vi "sub_UDP_Transmit.vi"(7 "UDP Config":T1, 8 "error in":errorcluster, 10 "Packets":string[](array[string]), 11 "UDP Network Connection in":refnum<k16>) -> (0 "error out":errorcluster, 3 "UDP Network Connection out":refnum<k16>)   [LabVIEW 2012]
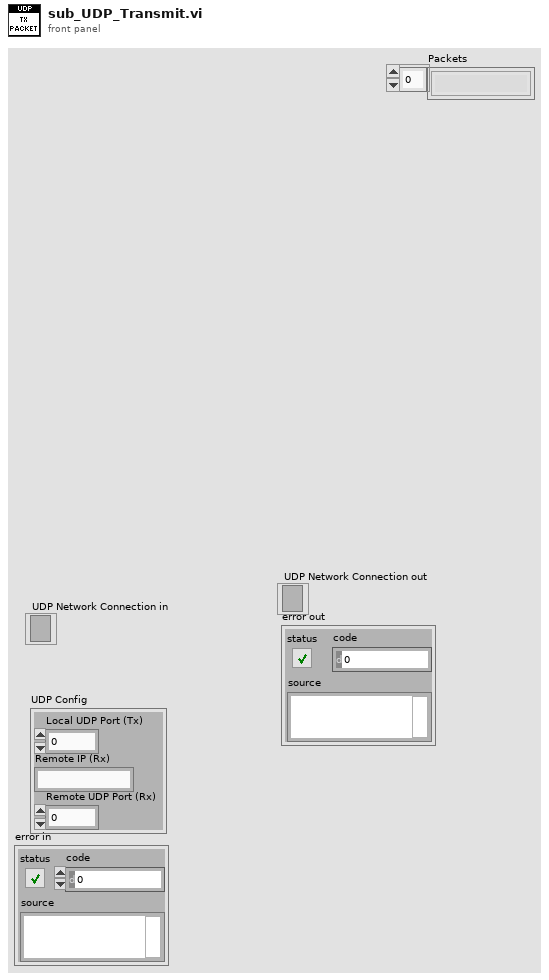
[diagram p1: front panel]
types:
  T1 = cluster{"Local UDP Port (Tx)":i16, "Remote IP (Rx)":string, "Remote UDP Port (Rx)":i16}
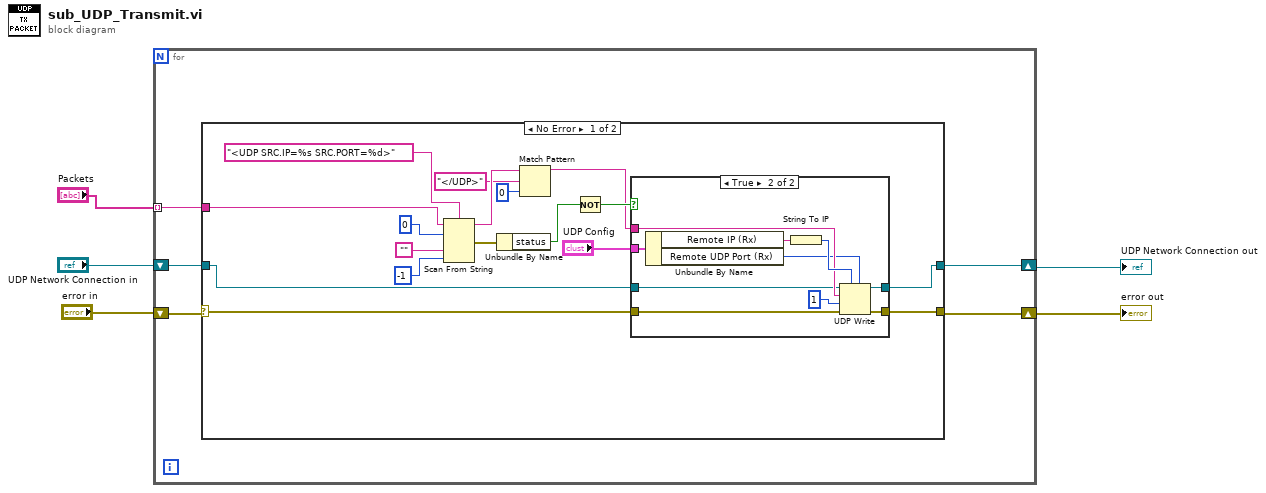
[diagram p0: block diagram]
diagram:
  n1 = for {
    shift-right: [w9] -> w4
    shift-left: "error in" -> [w7]
    shift-right: [w10] -> w5
    shift-left: "UDP Network Connection in" -> [w8]
    tunnel: "Packets" -> [w6] mode=indexing
    n2 = case shown="No Error" w7 {
      selector: w7 -> [w17 w41]
      tunnel: [w19 w40] -> w10
      tunnel: [w18 w41] -> w9
      tunnel: w8 -> [w16 w40]
      tunnel: w6 -> [w11 _]
      frame No Error {
        n3 = Scan From String(format string="<UDP SRC.IP=%s SRC.PORT=%d>", input string=w11, initial scan location=u32 0, default 1="", default 2=-1 ("default value 2")) -> (remaining string=w15:string, error out=w22:errorcluster)  [unwired: 3 in, 1 out]
        n4 = Unbundle By Name(w22) -> ("status"=w25:bool)
        n5 = Match Pattern(string=w15, regular expression="</UDP>", offset (0)=0) -> (before substring=w12:string)  [unwired: 3 out]
        n6 = Not(x=w25) -> (.not. x?=w26:bool)
        n7 = case shown="True" w26 {
          tunnel: w12 -> [_ w37]
          tunnel: "UDP Config" -> [_ w34]
          tunnel: w16 -> [w29 w36]
          tunnel: [w29 w32] -> w19
          tunnel: [w28 w31] -> w18
          tunnel: w17 -> [w28 w30]
          frame False {
          }
          frame True {
            n8 = Unbundle By Name(w34) -> ("Remote IP (Rx)"=w35:string, "Remote UDP Port (Rx)"=w33:i16)
            n9 = String To IP(1:w35) -> (0:w39:u32)
            n10 = UDP Write(address=w39, port or service name=w33, connection ID=w36, data in=w37, 8:w30, 9:1 ("timeout ms (25000)")) -> (error out=w31:errorcluster, 3:w32:refnum<k16>)
          }
        }
      }
      frame Error {
      }
    }
  }
  "UDP Network Connection out" <- w5
  "error out" <- w4
